vi "Memory.Pointer.Type Cast.vi"   [LabVIEW 2016, in "Memory Manager.lvlib" / "Memory.Pointer.lvclass"]
doc: "Moves bytes of data from the <b>src pointer</b> at <b>src offset</b> to the <b>dst pointer</b> at <b>dst offset</b> using the <b>byte order</b> specified. <b>src width</b> and <b>dst width</b> are used to determine how many bytes to move, as well as where the bytes should be read from/written to in memory.\n\nFor example, to type cast a DBL to a U16, src width would be 8 bytes and dst width would be 2 bytes."
uses:
  Memory.Pointer.lvclass
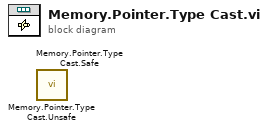
[diagram p0: block diagram]
diagram:
  n1 = call "Memory.Pointer.Type Cast.Unsafe.vi"() -> ()  [unwired: 13 in, 3 out]
  n2 = call "Memory.Pointer.Type Cast.Safe.vi"() -> ()  [unwired: 13 in, 3 out]
